vi "Configure.vi"(8 "error in (no error)":errorcluster, 10 "Msg in":T1, 11 "FakeCamera in":refnum<class "MoveDataFile.lvclass">) -> (0 "error out":errorcluster, 1 "new command":string, 2 "Msg out":T1, 3 "FakeCamera out":refnum<class "MoveDataFile.lvclass">)   [LabVIEW 2011, in "MoveDataFile.lvclass"]
uses:
  MoveDataFile.lvclass
  BaseDriver/DriverMsg.ctl
  MoveDataFile.lvclass/MoveDataFile.ctl
  shared/OnOffTypeDef.ctl
  BaseDriver/BaseDriver.lvclass
  shared/CompressAndUpdate(Poly)/CompressAndUpdate(String).vi
  shared/CompressAndUpdate(Poly)/CompressAndUpdate(Enum).vi
  shared/CompressAndUpdate(Poly)/CompressAndUpdate(Path).vi
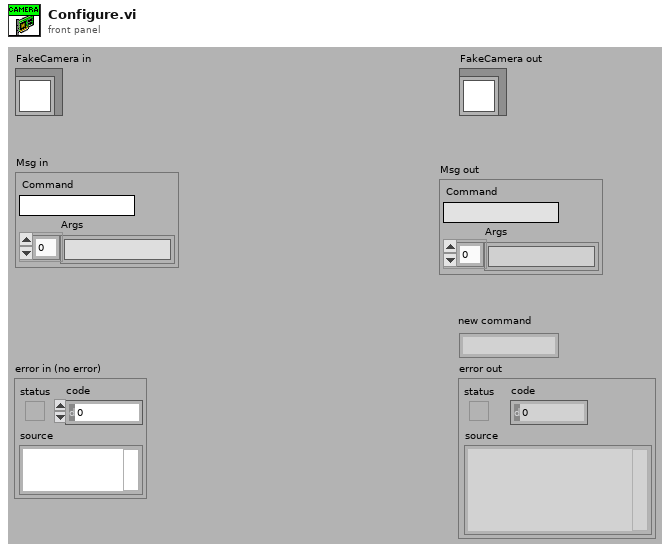
[diagram p1: front panel]
types:
  T1 = typedef "DriverMsg.ctl" = cluster{"Command":string, "Args":string[]}
  T2 = typedef "OnOffTypeDef.ctl" = enum16{"off", "on"}
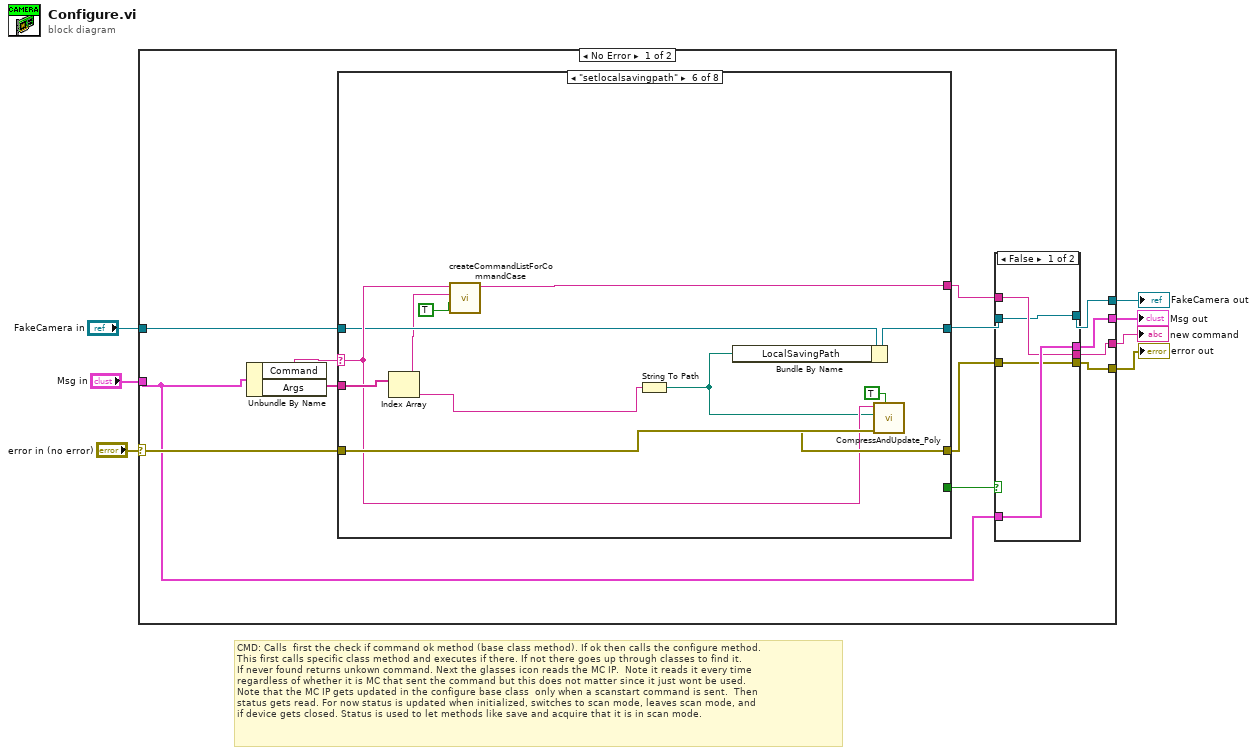
[diagram p0: block diagram]
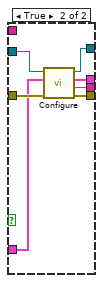
[diagram p2: hidden frame]
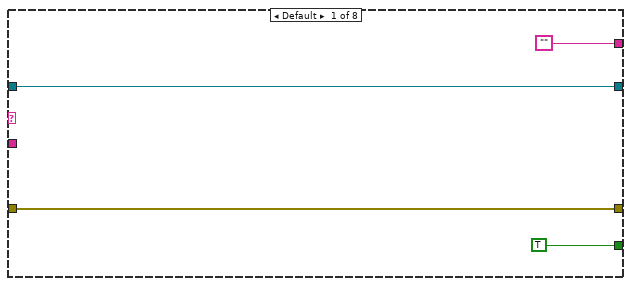
[diagram p3: hidden frame]
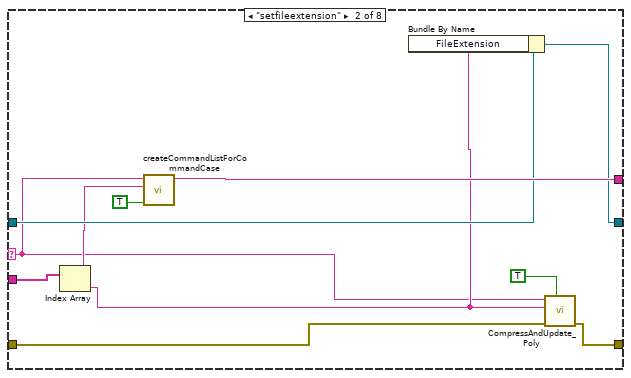
[diagram p4: hidden frame]
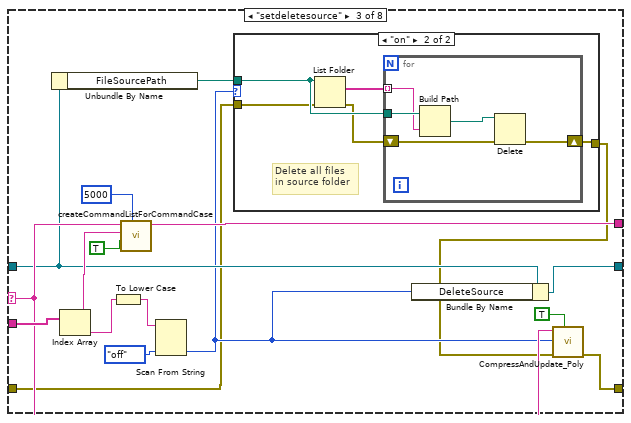
[diagram p5: hidden frame]
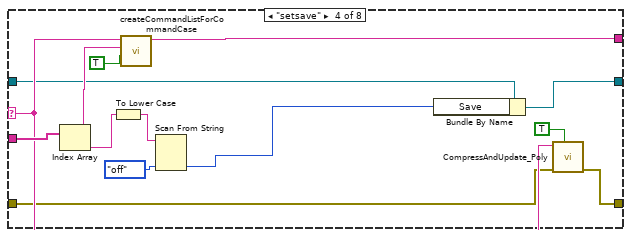
[diagram p7: hidden frame]
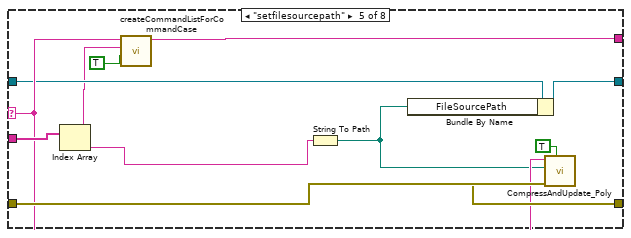
[diagram p8: hidden frame]
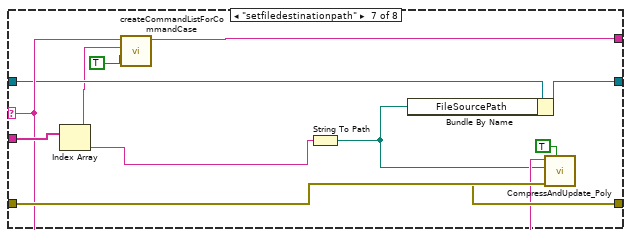
[diagram p9: hidden frame]
diagram:
  # "CMD: Calls  first the check if command ok method (base class method). If ok then calls the configure method.\nThis first calls specific class method and executes if there. If not there goes up through classes to find it.\nIf never found returns unkown command. Next the glasses icon reads the MC IP.  Note it reads it every time\nregardless of whether it is MC that sent the command but this does not matter since it just wont be used.\nNote that the MC IP gets updated in the configure base class  only when a scanstart command is sent.  Then\nstatus gets read. For now status is updated when initialized, switches to scan mode, leaves scan mode, and\nif device gets closed. Status is used to let methods like save and acquire that it is in scan mode."
  n1 = case shown="No Error" "error in (no error)" {
    selector: "error in (no error)" -> [w10 w123]
    tunnel: "FakeCamera in" -> [w9 w121]
    tunnel: [w17 w121] -> w4
    tunnel: [w15 w123] -> w2
    tunnel: "Msg in" -> [w8 w122]
    tunnel: [w13 w122] -> w7
    tunnel: [w11 _] -> w6
    frame No Error {
      n2 = Unbundle By Name(w8) -> ("Command"=w20:string, "Args"=w19:string[])
      n3 = case shown="\"setlocalsavingpath\"" w20 {
        selector: w20 -> [_ w36 w57 w81 w91 w102 w113 _]
        tunnel: w10 -> [w34 w43 w46 w73 w93 w104 w115 w119]
        tunnel: w19 -> [_ w41 w61 w85 w96 w107 w118 _]
        tunnel: w9 -> [w35 w40 w51 w75 w90 w101 w112 w120]
        tunnel: [w35 w39 w60 w84 w95 w106 w117 w120] -> w18
        tunnel: ["" ("Complete") w44 w59 w83 w94 w105 w116 _] -> w12
        tunnel: [w34 w42 w58 w82 w92 w103 w114 w119] -> w16
        tunnel: [TRUE _ _ _ _ _ _ _] -> w14
        frame Default {
        }
        frame "setfileextension" {
          n4 = Index Array(array=w41) -> (element=w37:string)  [unwired: 1 in]
          n5 = call "createCommandListForCommandCase.vi"("immediate Check (only once)"=TRUE, "setvalue"=w37, "command"=w36) -> ("new commands"=w44:string)  [unwired: 8 in]
          n6 = Bundle By Name(cluster=w40, "FileExtension"=w37) -> (w39:refnum<class "MoveDataFile.lvclass">)
          n7 = call-poly "CompressAndUpdate_Poly.vi"("force CVT update (false)"=TRUE ("force CVT update"), "error in"=w43, "String"=w37, "command or variable name"=w36) -> ("error out"=w42:errorcluster)  [unwired: 7 in]
        }
        frame "setdeletesource" {
          n8 = Unbundle By Name(w51) -> ("FileSourcePath"=w49:path)
          n9 = Index Array(array=w61) -> (element=w54:string)  [unwired: 1 in]
          n10 = To Lower Case(string=w54) -> (all lower case string=w53:string)
          n11 = call "createCommandListForCommandCase.vi"("timeout (optional)"=5000, "immediate Check (only once)"=TRUE, "setvalue"=w54, "command"=w57) -> ("new commands"=w59:string)  [unwired: 7 in]
          n12 = Scan From String(input string=w53, default 1=OnOffTypeDef."off" ("Settings.Trigger")) -> (output 1=w50:T2)  [unwired: 3 in, 3 out]
          n13 = case shown="\"on\"" w50 {
            tunnel: w49 -> [_ w66]
            tunnel: [w62 w64] -> w47
            tunnel: w46 -> [w62 w63]
            frame "off", Default {
            }
            frame "on" {
              # "Delete all files \nin source folder"
              n14 = List Folder(path=w66, error in=w63) -> (filenames=w67:string[], error out=w65:errorcluster)  [unwired: 2 in, 2 out]
              n15 = for {
                tunnel: w67 -> [w71] mode=indexing
                tunnel: w66 -> [w72]
                shift-right: [w69] -> w64
                shift-left: w65 -> [w68]
                n16 = Build Path(base path=w72, name or relative path=w71) -> (appended path=w70:path)
                n17 = Delete(path (use dialog)=w70, error in=w68) -> (error out=w69:errorcluster)  [unwired: 3 in, 2 out]
              }
            }
          }
          n18 = Bundle By Name(cluster=w51, "DeleteSource"=w50) -> (w60:refnum<class "MoveDataFile.lvclass">)
          n19 = call-poly "CompressAndUpdate_Poly.vi"("force CVT update (false)"=TRUE ("force CVT update"), "error in"=w47, "enum variant"=w50, "command or variable name"=w57) -> ("error out"=w58:errorcluster)  [unwired: 7 in]
        }
        frame "setsave" {
          n20 = Index Array(array=w85) -> (element=w78:string)  [unwired: 1 in]
          n21 = To Lower Case(string=w78) -> (all lower case string=w77:string)
          n22 = call "createCommandListForCommandCase.vi"("immediate Check (only once)"=TRUE, "setvalue"=w78, "command"=w81) -> ("new commands"=w83:string)  [unwired: 8 in]
          n23 = Scan From String(input string=w77, default 1=OnOffTypeDef."off" ("Settings.Trigger")) -> (output 1=w74:T2)  [unwired: 3 in, 3 out]
          n24 = Bundle By Name(cluster=w75, "Save"=w74) -> (w84:refnum<class "MoveDataFile.lvclass">)
          n25 = call-poly "CompressAndUpdate_Poly.vi"("force CVT update (false)"=TRUE ("force CVT update"), "error in"=w73, "command or variable name"=w81) -> ("error out"=w82:errorcluster)  [unwired: 8 in]
        }
        frame "setfilesourcepath" {
          n26 = Index Array(array=w96) -> (element=w88:string)  [unwired: 1 in]
          n27 = call "createCommandListForCommandCase.vi"("immediate Check (only once)"=TRUE, "setvalue"=w88, "command"=w91) -> ("new commands"=w94:string)  [unwired: 8 in]
          n28 = String To Path(string=w88) -> (path=w87:path)
          n29 = Bundle By Name(cluster=w90, "FileSourcePath"=w87) -> (w95:refnum<class "MoveDataFile.lvclass">)
          n30 = call-poly "CompressAndUpdate_Poly.vi"("force CVT update (false)"=TRUE ("force CVT update"), "error in"=w93, "Path"=w87, "command or variable name"=w91) -> ("error out"=w92:errorcluster)  [unwired: 7 in]
        }
        frame "setlocalsavingpath" {
          n31 = Index Array(array=w107) -> (element=w99:string)  [unwired: 1 in]
          n32 = call "createCommandListForCommandCase.vi"("immediate Check (only once)"=TRUE, "setvalue"=w99, "command"=w102) -> ("new commands"=w105:string)  [unwired: 8 in]
          n33 = String To Path(string=w99) -> (path=w98:path)
          n34 = Bundle By Name(cluster=w101, "LocalSavingPath"=w98) -> (w106:refnum<class "MoveDataFile.lvclass">)
          n35 = call-poly "CompressAndUpdate_Poly.vi"("force CVT update (false)"=TRUE ("force CVT update"), "error in"=w104, "Path"=w98, "command or variable name"=w102) -> ("error out"=w103:errorcluster)  [unwired: 7 in]
        }
        frame "setfiledestinationpath" {
          n36 = Index Array(array=w118) -> (element=w110:string)  [unwired: 1 in]
          n37 = call "createCommandListForCommandCase.vi"("immediate Check (only once)"=TRUE, "setvalue"=w110, "command"=w113) -> ("new commands"=w116:string)  [unwired: 8 in]
          n38 = String To Path(string=w110) -> (path=w109:path)
          n39 = Bundle By Name(cluster=w112, "FileSourcePath"=w109) -> (w117:refnum<class "MoveDataFile.lvclass">)
          n40 = call-poly "CompressAndUpdate_Poly.vi"("force CVT update (false)"=TRUE ("force CVT update"), "error in"=w115, "Path"=w109, "command or variable name"=w113) -> ("error out"=w114:errorcluster)  [unwired: 7 in]
        }
        frame "Abort" {
        }
      }
      n41 = case shown="False" w14 {
        tunnel: w18 -> [w22 w31]
        tunnel: [w22 w30] -> w17
        tunnel: [w23 w29] -> w11
        tunnel: w16 -> [w21 w28]
        tunnel: [w21 w27] -> w15
        tunnel: w8 -> [w24 w26]
        tunnel: [w24 w25] -> w13
        tunnel: w12 -> [w23 _]
        frame False {
        }
        frame True {
          n42 = call-parent "Configure.vi"("error in (no error)"=w28, "Msg in"=w26, "BaseDriver in"=w31) -> ("error out"=w27:errorcluster, "new command"=w29:string, "Msg out"=w25:T1, "BaseDriver out"=w30:refnum<class "MoveDataFile.lvclass">)  [unwired: 5 in]
        }
      }
    }
    frame Error {
    }
  }
  "error out" <- w2
  "FakeCamera out" <- w4
  "new command" <- w6
  "Msg out" <- w7
